vi "数字输出_连续.vi"() -> ()   [LabVIEW 2013]
doc: "This example demonstrates how to read values from a digital input port."
uses:
  <userlib>/ArtDAQ/_SubVI/ArtDAQ_CreateDOChan.vi
  <userlib>/ArtDAQ/_SubVI/ArtDAQ_CfgSampClkTiming.vi
  <userlib>/ArtDAQ/_SubVI/ArtDAQ_Write Digital Bool NChan NSamp.vi
  <userlib>/ArtDAQ/_SubVI/ArtDAQ_CfgDigEdgeStartTrig.vi
panel:
  in  "?":bool[][](array[boolean])=[[TRUE, FALSE, TRUE, FALSE], [FALSE, FALSE, FALSE, FALSE], [FALSE, TRUE, FALSE, TRUE]]
  out "错误输出":errorcluster
  in  "触发模式":enum32{"无触发", "数字边沿"}(tab)
  in  "有效边沿":i32(ring)=10280 items=["上升"=10280, "下降"=10171]
  in  "触发源":string
  in  "每通道采样数":i32=4
  in  "采样速率":dbl=10.0
  in  "时钟源":string="/Dev1/PFI0"
  in  "?":bool
  in  "端口":string="Dev1/port0/line0:2"
  # "通道属性"
  # "定时"
  # "触发"
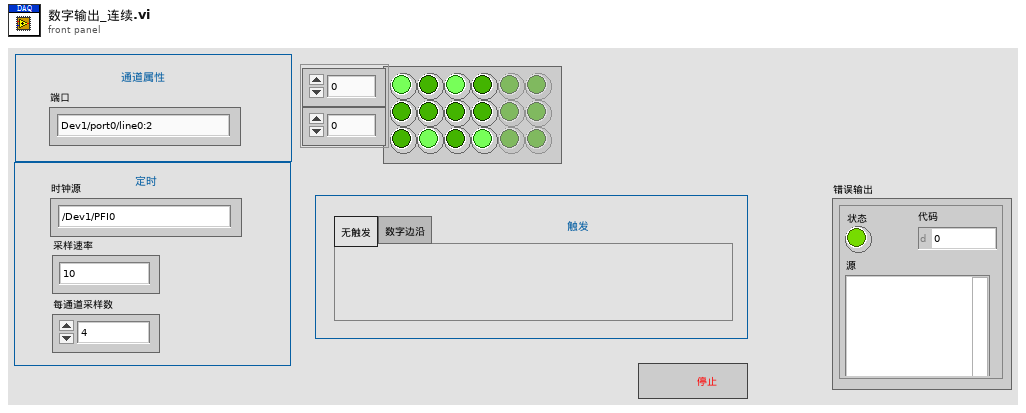
[diagram p1: front panel]
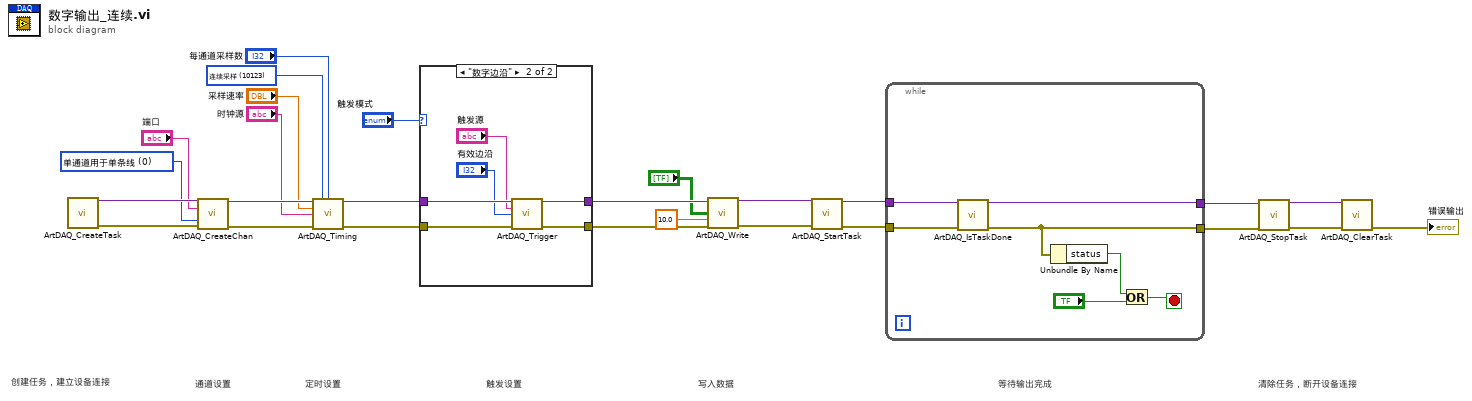
[diagram p0: block diagram]
diagram:
  w12 = 10123 items=["有限点采样"=10178, "连续采样"=10123] ("SampleMode")
  w17 = 0 items=["单通道用于单条线", "单通道用于所有线"] ("Line Grouping")
  # "清除任务，断开设备连接"
  # "等待输出完成"
  # "写入数据"
  # "触发设置"
  # "定时设置"
  # "通道设置"
  # "创建任务，建立设备连接"
  n1 = call <userlib>:"ArtDAQ_CreateTask.vi"() -> ("任务句柄"=w26:variant, "错误输出"=w25:errorcluster)  [unwired: 14 in]
  n2 = call-poly <userlib>:"ArtDAQ_CreateChan.vi"("任务句柄"=w26, "线"="端口", "线分组"=w17, "错误输入"=w25) -> ("任务句柄"=w15:variant, "错误输出"=w16:errorcluster)  [unwired: 10 in]
  n3 = call-poly <userlib>:"ArtDAQ_Timing.vi"("任务句柄"=w15, "采样模式"=w12, "每通道采样数"="每通道采样数", "采样率"="采样速率", "源"="时钟源", "错误输入"=w16) -> ("任务句柄"=w10:variant, "错误输出"=w9:errorcluster)  [unwired: 8 in]
  n4 = case shown="\"数字边沿\"" "触发模式" {
    tunnel: w10 -> [w28 w34]
    tunnel: w9 -> [w27 w33]
    tunnel: [w28 w32] -> w4
    tunnel: [w27 w31] -> w7
    frame "无触发", Default {
    }
    frame "数字边沿" {
      n5 = call-poly <userlib>:"ArtDAQ_Trigger.vi"("任务句柄"=w34, "触发源"="触发源", "边沿"="有效边沿", "错误输入"=w33) -> ("任务句柄"=w32:variant, "错误输出"=w31:errorcluster)  [unwired: 10 in]
    }
  }
  n6 = call-poly <userlib>:"ArtDAQ_Write.vi"("任务句柄"=w4, "数据"="?", "超时s"=10.0 ("Timeout"), "错误输入"=w7) -> ("任务句柄"=w5:variant, "错误输出"=w6:errorcluster)  [unwired: 9 in, 1 out]
  n7 = call <userlib>:"ArtDAQ_StartTask.vi"("任务句柄"=w5, "错误输入"=w6) -> ("任务句柄"=w24:variant, "错误输出"=w23:errorcluster)  [unwired: 12 in]
  n8 = while {
    tunnel: w24 -> [w41]
    tunnel: w23 -> [w40]
    tunnel: [w39] -> w22
    tunnel: [w38] -> w21
    stop <- w35 stop-if-true
    n9 = call <userlib>:"ArtDAQ_IsTaskDone.vi"("任务句柄"=w41, "错误输入"=w40) -> ("任务句柄"=w39:variant, "错误输出"=w38:errorcluster)  [unwired: 11 in, 1 out]
    n10 = Unbundle By Name(w38) -> ("status"=w37:bool)
    n11 = Or(x=w37, y="?") -> (x .or. y?=w35:bool)
  }
  n12 = call <userlib>:"ArtDAQ_StopTask.vi"("任务句柄"=w22, "错误输入"=w21) -> ("任务句柄"=w19:variant, "错误输出"=w20:errorcluster)  [unwired: 12 in]
  n13 = call <userlib>:"ArtDAQ_ClearTask.vi"("任务句柄"=w19, "错误输入"=w20) -> ("错误输出"=→"错误输出":errorcluster)  [unwired: 13 in]
